vi "Defense_Int_to_Enum.vi"(1 "Defense":T1) -> (0 "Defense":T1)   [LabVIEW 2015]
uses:
  Auton Defenses Enum.ctl
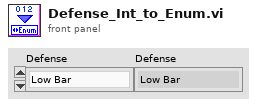
[diagram p1: front panel]
types:
  T1 = typedef "Auton Defenses Enum.ctl" = enum16{"Low Bar", "None", "Portcullis", "CDF", "Moat", "Ramparts", "Drawbridge", "Sally Port", "Rock Wall", "Rough Terrain"}
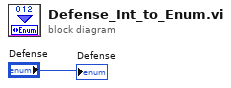
[diagram p0: block diagram]
diagram:
  "Defense" <- "Defense"
